vi "user process.vi"(8 "error in":errorcluster, 11 "Parameters to process":T2) -> (0 "error out":errorcluster, 3 "Results from processing":T1)   [LabVIEW 2017, in "AppStateMachine runtime.lvclass"]
uses:
  AppStateMachine runtime.lvclass
  parameter user data.ctl
  result user data.ctl
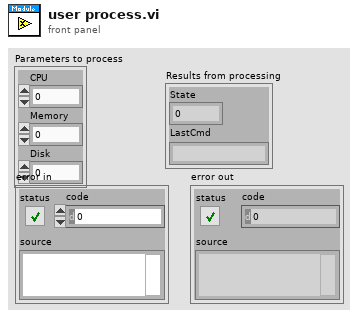
[diagram p1: front panel]
types:
  T1 = typedef "AppStateMachine runtime.lvclass/result user data.ctl" = cluster{"State":u16, "LastCmd":string}
  T2 = typedef "AppStateMachine runtime.lvclass/parameter user data.ctl" = cluster{"CPU":dbl, "Memory":dbl, "Disk":dbl}
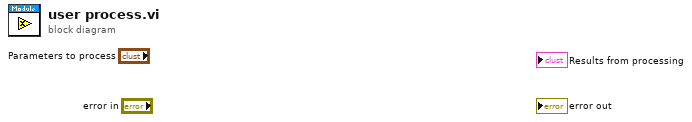
[diagram p0: block diagram]
diagram:
